vi "Clocks.vi"(2 "error in (no error)":errorcluster, 3 "Enum":enum16{"Reset", "Increment", "Get"}(ring)=enum."Get") -> (0 "error out":errorcluster, 1 "Clock":u64)   [LabVIEW 2023]
uses:
  <vilib>/rvi/Emulation/niFpgaGetClockAttributes.vi
  <vilib>/rvi/Emulation/niFpgaSctlEmulationGetInTimedLoop.vi
  <vilib>/rvi/Emulation/niFpgaEmulationReportErrorSimple.vi
  <vilib>/rvi/Emulation/niFpgaCriticalErrorInLSC.vi
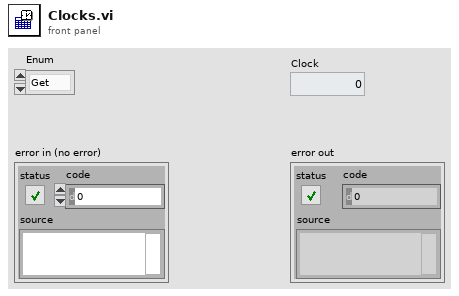
[diagram p1: front panel]
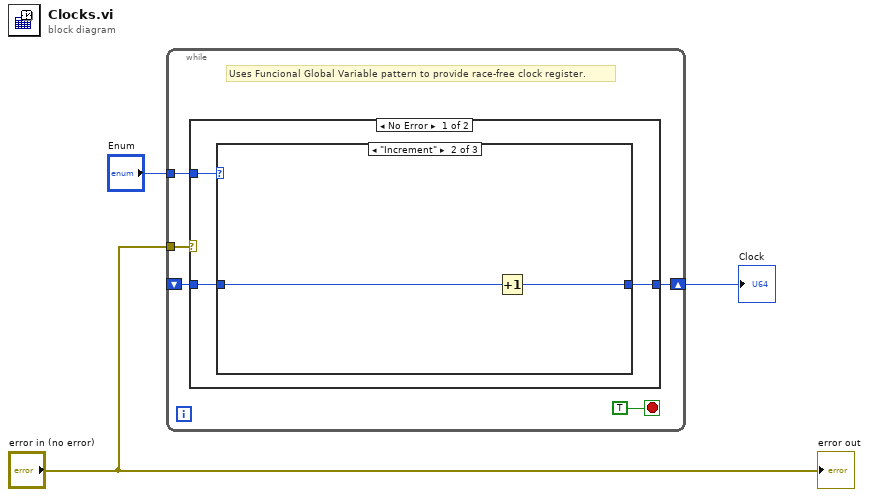
[diagram p0: block diagram]
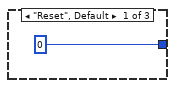
[diagram p2: hidden frame]
diagram:
  n1 = while {
    tunnel: "Enum" -> [w7]
    tunnel: "error in (no error)" -> [w6]
    shift-right: [w5] -> w1
    shift-left: _ -> [w4]
    stop <- TRUE stop-if-true
    # "Uses Funcional Global Variable pattern to provide race-free clock register."
    n2 = case shown="No Error" w6 {
      tunnel: w7 -> [w11 _]
      tunnel: [w10 w16] -> w5
      tunnel: w4 -> [w9 w16]
      frame No Error {
        n3 = case shown="\"Increment\"" w11 {
          tunnel: [u64 0 w13 w15] -> w10
          tunnel: w9 -> [_ w14 w15]
          frame "Reset", Default {
          }
          frame "Increment" {
            n4 = Increment(x=w14) -> (x+1=w13:u64)
          }
          frame "Get" {
          }
        }
      }
      frame Error {
      }
    }
  }
  "Clock" <- w1
  "error out" <- "error in (no error)"
